vi "RTInit.vi"(8 "error in (no error)":errorcluster) -> (0 "error out":errorcluster, 3 "FPGA VI Reference Out":refnum<k20>)   [LabVIEW 2016]
uses:
  <vilib>/FPGAPlugInAG/cRIO-9066/niLvFpga_Open_cRIO-9066.vi
  <vilib>/rvi/interface/common/dynamic/niFpgaDynamicAddResources.vi
  <vilib>/rvi/interface/nirviOpenFPGA/nirviOpenFPGA.xnode
  FPGA Bitfiles/FEM_FPGA_bitfile.lvbitx
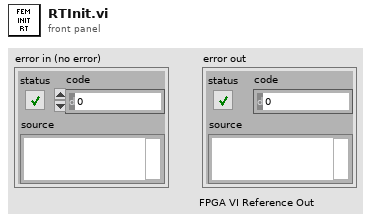
[diagram p1: front panel]
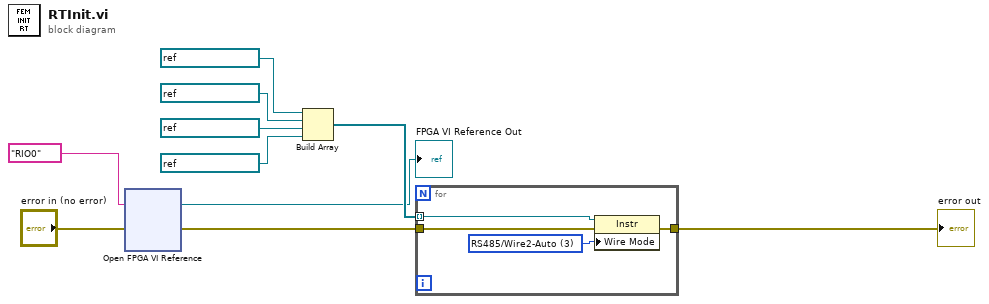
[diagram p0: block diagram]
diagram:
  n1 = xnode "Open FPGA VI Reference"("error in"="error in (no error)", "resource name"=tag "RIO0") -> ("FPGA VI Reference Out"=→"FPGA VI Reference Out":refnum<k20>, "error out"=w3:errorcluster)
  n2 = Build Array(refnum<visa-resource-name> "ASRL2::INSTR" ("VISA resource name"), refnum<visa-resource-name> "ASRL3::INSTR" ("VISA resource name"), refnum<visa-resource-name> "ASRL4::INSTR" ("VISA resource name"), refnum<visa-resource-name> "ASRL5::INSTR" ("VISA resource name")) -> (w10:refnum<visa-resource-name>[])
  n3 = for {
    tunnel: w10 -> [w12] mode=indexing
    tunnel: w3 -> [w14]
    tunnel: [w13] -> w2
    w11 = i16 3 items=["Unknown"=-1, "RS485/Wire4"=0, "RS485/Wire2-EchoDTR"=1, "RS485/Wire2-CtrlDTR"=2, "RS485/Wire2-Auto"=3, "RS232/DTE"=128, "RS232/DCE"=129, "RS232/Auto"=130] ("Serial Settings:Wire Mode")
    n4 = property class="Instr"(reference=w12, error in=w14, "Wire Mode"=w11) -> (error out=w13:errorcluster)  [unwired: 1 out]
  }
  "error out" <- w2
